vi "SnapGreyImage.vi"(3 "error in (no error)":errorcluster, 5 "QT Ref In":T1) -> (0 "error out":errorcluster={"status"=TRUE, "code"=-43, "source"=""}, 1 "Image Out":T2 {"Dialogs" format="%.0b"}, 2 "QT Ref Out":T1)   [LabVIEW 2024]
doc: "This VI takes an 8 bit grey scale image from a live camera."
uses:
  <userlib>/ImageProcessing/QTLIB_2595_LV86/QT_Ref.ctl
  <userlib>/ImageProcessing/QTLIB_2595_LV86/QT_Image.ctl
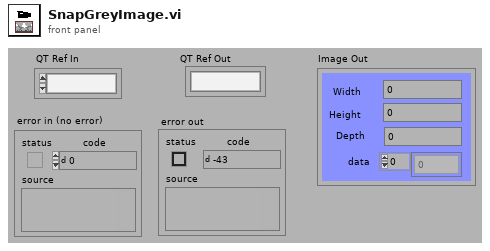
[diagram p1: front panel]
types:
  T1 = typedef "QT_Ref.ctl" = refnum<k1>
  T2 = typedef "QT_Image.ctl" = cluster{"Width":i32, "Height":i32, "Depth":i32, "data":u8[], "Compressed data":u8[], "Color table":u32[], "Duration":i32, "Options":i32, "Timestamp":i32, "ID":i32, "Reserved":i32, "Dialogs":u32}
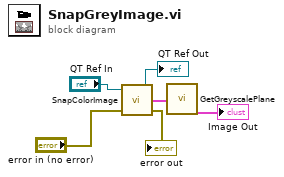
[diagram p0: block diagram]
diagram:
  n1 = call <userlib>:"SnapColorImage.vi"("error in (no error)"="error in (no error)", "QT Ref In"="QT Ref In") -> ("error out"=→"error out":errorcluster, "Image Out"=w6:T2, "QT Ref Out"=→"QT Ref Out":T1)  [unwired: 1 out]
  n2 = call <userlib>:"GetGreyscalePlane.vi"("Image In"=w6) -> ("Greyscale  Out"=→"Image Out":T2)
